vi "Elait_HEXstring_READ_BUFFER.vi"(8 "error in":T6, 11 "DriverConnect in":T1={"InterfaceType"=enum."VISA", "OpenedSession"="", "InterfaceSettings"={"Interface"=enum."RS232", "EOS 4 read"=enum."LF (\\n)", "EOS 4 write"=enum."LF (\\n)", "TMO, ms"=10000, "Sett"=variant(cluster{"Baud Rate":u32, "Data Bits":u16, "Parity":u16, "Stop Bits":u16, "Flow Control":u16, "Eho":bool} {"Baud Rate"=75, "Data Bits"=0, "Parity"=0, "Stop Bits"=0, "Flow Control"=0, "Eho"=FALSE})}}) -> (0 "error out":T6, 3 "DriverConnect out":T1={"InterfaceType"=enum."VISA", "OpenedSession"="", "InterfaceSettings"={"Interface"=enum."RS232", "EOS 4 read"=enum."LF (\\n)", "EOS 4 write"=enum."LF (\\n)", "TMO, ms"=10000, "Sett"=variant(cluster{"Baud Rate":u32, "Data Bits":u16, "Parity":u16, "Stop Bits":u16, "Flow Control":u16, "Eho":bool} {"Baud Rate"=75, "Data Bits"=0, "Parity"=0, "Stop Bits"=0, "Flow Control"=0, "Eho"=FALSE})}}, 5 "String from device out":string)   [LabVIEW 2018]
uses:
  MOKO_LabViewLibrary/MokoLowLevel/MokoLowLovelControl/MLLC_Error.ctl
  MOKO_LabViewLibrary/MokoLowLevel/MokoLowLovelControl/MLLC_ConnectCluster.ctl
  MOKO_LabViewLibrary/MokoLowLevel/MokoLowLovelControl/MLLC_InterfaceType.ctl
  MOKO_LabViewLibrary/MokoLowLevel/MokoLowLovelControl/MLLC_OpenedSession.ctl
  MOKO_LabViewLibrary/MokoLowLevel/MokoLowLovelControl/MLLC_InterfaceSettings.ctl
  MOKO_LabViewLibrary/MokoLowLevel/MokoLowLovelControl/MLLC_InterfaceKind.ctl
  MOKO_LabViewLibrary/MokoLowLevel/MokoLowLovelControl/MLLC_Rs232Settings.ctl
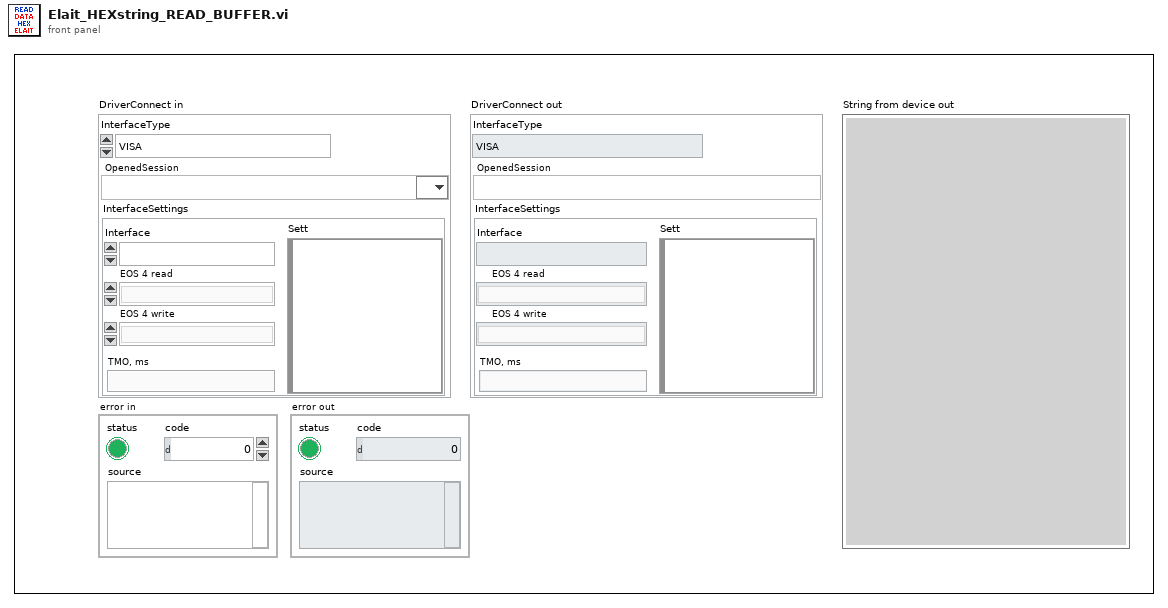
[diagram p1: front panel]
types:
  T1 = typedef "MLLC_ConnectCluster.ctl" = cluster{"InterfaceType":T2, "OpenedSession":T3, "InterfaceSettings":T4}
  T2 = typedef "MLLC_InterfaceType.ctl" = enum16{"VISA", "Prologix USB-GPIB"}
  T3 = typedef "MLLC_OpenedSession.ctl" = refnum<visa-resource-name>
  T4 = typedef "MLLC_InterfaceSettings.ctl" = cluster{"Interface":T5, "EOS 4 read":enum16{"Default (=EOS 4 write)", "CR (\\r)", "LF (\\n)", "None"}, "EOS 4 write":enum16{"CR+LF (\\r\\n)", "CR (\\r)", "LF (\\n)", "None"}, "TMO, ms":i32, "Sett":variant}
  T5 = typedef "MLLC_InterfaceKind.ctl" = enum16{"RS232", "GPIB", "USB", "Ethernet", "another"}
  T6 = typedef "MLLC_Error.ctl" = errorcluster
  T7 = typedef "MLLC_Rs232Settings.ctl" = cluster{"Baud Rate":u32, "Data Bits":u16, "Parity":u16, "Stop Bits":u16, "Flow Control":u16, "Eho":bool, "Address":dbl}
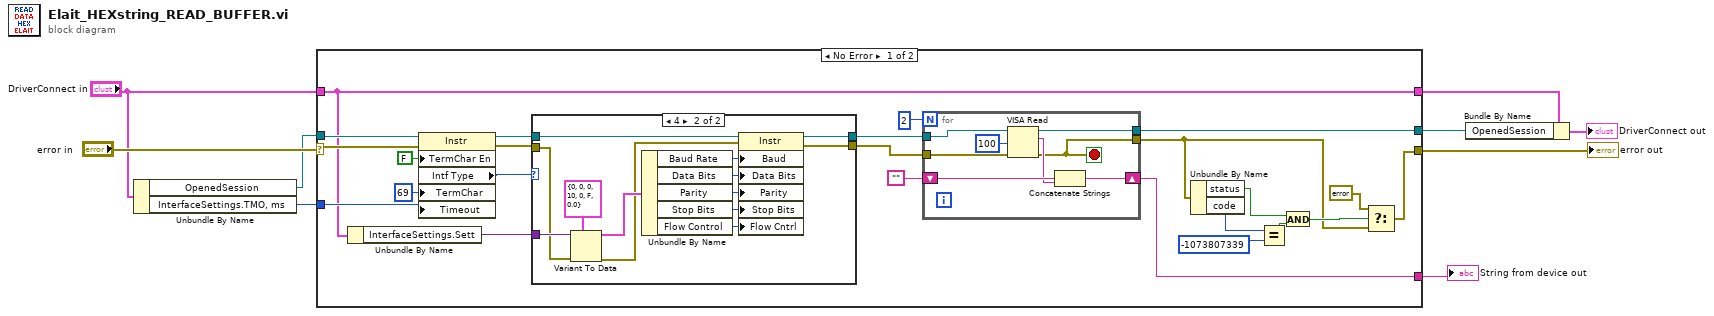
[diagram p0: block diagram]
diagram:
  n1 = Unbundle By Name("DriverConnect in") -> ("OpenedSession"=w4:T3, "InterfaceSettings.TMO, ms"=w6:i32)
  n2 = case shown="No Error" "error in" {
    selector: "error in" -> [w26 w58]
    tunnel: [w18 _] -> w9
    tunnel: w4 -> [w25 w57]
    tunnel: [w32 w58] -> w8
    tunnel: [w19 w57] -> w3
    tunnel: "DriverConnect in" -> [w10 w59]
    tunnel: [w10 w59] -> w2
    tunnel: w6 -> [w11 _]
    frame No Error {
      n3 = Unbundle By Name(w10) -> ("InterfaceSettings.Sett"=w22:variant)
      n4 = property class="Instr"(reference=w25, error in=w26, "TermChar En"=FALSE ("Message Based Settings:Termination Character Enable"), "TermChar"=u8 69 ("Message Based Settings:Termination Character"), "Timeout"=w11) -> (reference out=w24:T3, error out=w23:errorcluster, "Intf Type"=w21:u16)
      n5 = case shown="4" w21 {
        tunnel: [w43 w53] -> w14
        tunnel: w24 -> [w43 w54]
        tunnel: [w42 w45] -> w13
        tunnel: w23 -> [w42 w55]
        tunnel: w22 -> [_ w56]
        frame 0, Default {
        }
        frame 4 {
          n6 = Variant To Data(error in=w55, type=T7 {"Baud Rate"=0, "Data Bits"=0, "Parity"=0, "Stop Bits"=10, "Flow Control"=0, "Eho"=FALSE, "Address"=0.0} ("Cluster"), Variant=w56) -> (data=w51:T7, error out=w44:errorcluster)
          n7 = Unbundle By Name(w51) -> ("Baud Rate"=w50:u32, "Data Bits"=w46:u16, "Parity"=w47:u16, "Stop Bits"=w48:u16, "Flow Control"=w49:u16)
          n8 = property class="Instr"(reference=w54, error in=w44, "Baud"=w50, "Data Bits"=w46, "Parity"=w47, "Stop Bits"=w48, "Flow Cntrl"=w49) -> (reference out=w53:T3, error out=w45:errorcluster)
        }
      }
      n9 = for {
        N: 2 ("length (rest)") -> [_]
        shift-right: [w37] -> w18
        shift-left: "" -> [w36]
        tunnel: w14 -> [w40]
        tunnel: w13 -> [w39]
        tunnel: [w34] -> w20
        tunnel: [w38] -> w19
        stop <- w34 stop-if-true
        n10 = VISA Read(VISA resource name=w40, byte count=u32 100, error in (no error)=w39) -> (VISA resource name out=w38:T3, read buffer=w35:string, error out=w34:errorcluster)  [unwired: 1 out]
        n11 = Concatenate Strings(w36, w35) -> (w37:string)
      }
      n12 = Unbundle By Name(w20) -> ("status"=w28:bool, "code"=w31:i32)
      n13 = Equal?(x=w31, y=-1073807339) -> (x = y?=w29:bool)
      n14 = And(x=w28, y=w29) -> (x .and. y?=w27:bool)
      n15 = Select(t=errorcluster {"status"=FALSE, "code"=0, "source"=""} ("error IO"), s=w27, f=w20) -> (s? t:f=w32:errorcluster)
    }
    frame Error {
    }
  }
  "String from device out" <- w9
  "error out" <- w8
  n16 = Bundle By Name(cluster=w2, "OpenedSession"=w3) -> (→"DriverConnect out":T1)
